vi "Periodic Tasks.vi"(8 "error in":errorcluster) -> ()   [LabVIEW 2018]
doc: "This VI runs in parallel to other robot code. It can contain as many user-defined periodic loops as you need. These can carry out PID or other sorts of timed response."
uses:
  <vilib>/Rock Robotics/WPI/DriverStation/WPI_DriverStationRobotMode2.ctl
  Robot Global Data.vi
  <vilib>/Rock Robotics/Network Tables/NT Read String.vi
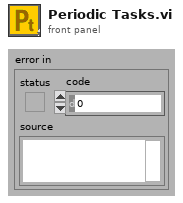
[diagram p1: front panel]
types:
  T1 = typedef "WPI_DriverStationRobotMode2.ctl" = enum16{"Autonomous Disabled", "Autonomous Enabled", "Teleop Disabled", "Teleop Enabled", "Disconnected", "Finish", "Test Disabled", "Test Enabled", "Emergency Stopped"}
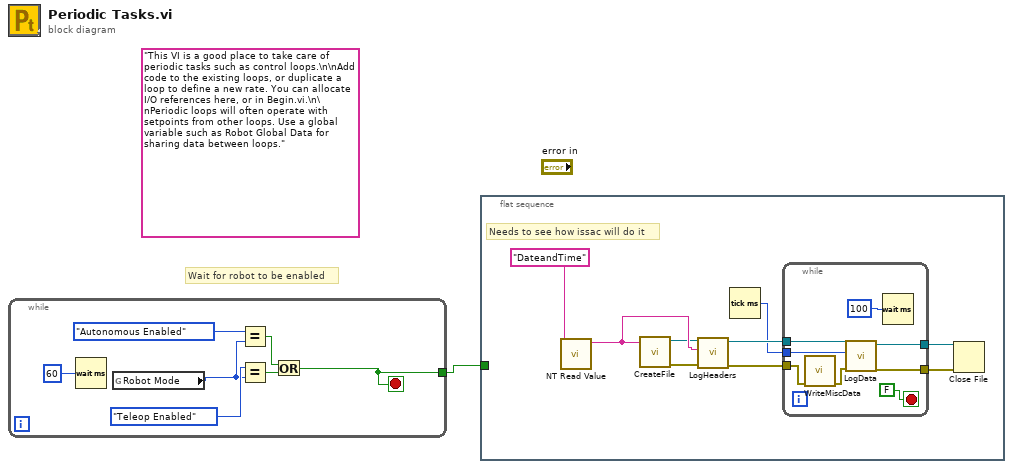
[diagram p0: block diagram]
diagram:
  (unwired) "This VI is a good place to take care of periodic tasks such as control loops.\n\nAdd code to the existing loops, or duplicate a loop to define a new rate. You can allocate I/O references here, or in Begin.vi.\n\nPeriodic loops will often operate with setpoints from other loops. Use a global variable such as Robot Global Data for sharing data between loops."
  # "Wait for robot to be enabled"
  n1 = while {
    tunnel: [w3] -> w1
    stop <- w3 stop-if-true
    n2 = Wait (ms)(milliseconds to wait=u32 60) -> ()  [unwired: 1 out]
    n3 = global read "Robot Global Data.vi" "Robot Mode"() -> (w2:T1)
    n4 = Equal?(x=WPI_DriverStationRobotMode2."Autonomous Enabled", y=w2) -> (x = y?=w5:bool)
    n5 = Equal?(x=WPI_DriverStationRobotMode2."Teleop Enabled", y=w2) -> (x = y?=w6:bool)
    n6 = Or(x=w5, y=w6) -> (x .or. y?=w3:bool)
  }
  n7 = flat-sequence {
    tunnel: w1 -> [_]
    frame #0 {
      # "Needs to see how issac will do it"
      n8 = call-poly <vilib>:"NT Read Value.vi"("Name"="DateandTime") -> ("String"=w17:string)  [unwired: 9 in, 1 out]
      n9 = call "CreateFile.vi"("Date/time"=w17) -> ("error out"=w14:errorcluster, "Byte Stream File out"=w16:refnum<file>)  [unwired: 9 in]
      n10 = call "LogHeaders.vi"("error in"=w14, "Date and Time"=w17, "refnum in"=w16) -> ("error out"=w13:errorcluster, "refnum out"=w15:refnum<file>)  [unwired: 7 in]
      n11 = Tick Count (ms)() -> (millisecond timer value=w12:u32)
      n12 = while {
        tunnel: w15 -> [w25]
        tunnel: w13 -> [w19]
        tunnel: w12 -> [w22]
        tunnel: [w21] -> w11
        tunnel: [w20] -> w10
        stop <- FALSE stop-if-true
        n13 = call "WriteMiscData.vi"("error in (no error)"=w19) -> ("error out"=w18:errorcluster)  [unwired: 10 in]
        n14 = call "LogData.vi"("error in (no error)"=w18, "Start time"=w22, "Refmum"=w25) -> ("error out"=w20:errorcluster, "Byte Stream File out"=w21:refnum<file>)  [unwired: 7 in]
        n15 = Wait (ms)(milliseconds to wait=u32 100) -> ()  [unwired: 1 out]
      }
      n16 = Close File(refnum=w11, error in=w10) -> ()  [unwired: 2 out]
    }
  }
